vi "Autonomous Independent.vi"   [LabVIEW 2013]
doc: "This VI is called when autonomous begins, and will automatically be terminated when autonomous ends. You can carry out timed or sensor driven robot movement independently without needing to return to the caller."
uses:
  <vilib>/Rock Robotics/WPI/Solenoid/WPI_SolenoidValue.ctl
  Robot Global Data.vi
  <vilib>/Rock Robotics/WPI/RobotDrive/WPI_RobotDriveGetSetRefNum.vi
  <vilib>/Rock Robotics/WPI/Solenoid/WPI_SolenoidSetEnum.vi
  <vilib>/Rock Robotics/WPI/RobotDrive/WPI_RobotDriveArcadeDrive_Standard(NoSaturation).vi
  <vilib>/Rock Robotics/WPI/Solenoid/Deprecated/WPI_SolenoidGetBool.vi
  <vilib>/Rock Robotics/WPI/Joystick/WPI_JoystickGetSetRefNum.vi
panel:
  # "Be sure to right-click and choose Data Operations>>Make Current Value default if you want to save the array values with the VI"
types:
  T1 = typedef "WPI_JoystickDevRef.ctl" = cluster{"Device":T2}
  T2 = typedef "WPI_JoystickDeviceEnum.ctl" = enum16{"USB 1", "USB 2", "USB 3", "USB 4", "Kinect 1", "Kinect 2"}
  T3 = typedef "WPI_MotorControlDeviceRef.ctl" = cluster{"DeviceStatus":errorcluster, "Type":enum16{"PWM", "CAN"}, "PWM":cluster{"Digital Module":T4, "PWM Channel":T5, "DeadBand":T6}, "CAN":cluster{"Device Number":u8, "Control Mode":T7, "Semaphore":T8, "Max Vout":dbl}, "Invert":bool, "TransformRef":T9, "InvTransformRef":T9}
  T4 = typedef "FPGA_TypedefDigitalModule.ctl" = enum16{"Digital Module 1", "Digital Module 2"}
  T5 = typedef "FPGA_DIOPWMChannel.ctl" = enum8{"PWM 1", "PWM 2", "PWM 3", "PWM 4", "PWM 5", "PWM 6", "PWM 7", "PWM 8", "PWM 9", "PWM 10", "Invalid"}
  T6 = typedef "WPI_PWMDeadband.ctl" = cluster{"Name":string, "maxPositivePwm":i32, "minPositivePwm":i32, "centerPwm":i32, "maxNegativePwm":i32, "minNegativePwm":i32, "angularRange":u16}
  T7 = typedef "WPI_CANJaguar_ControlMode.ctl" = enum8{"Percent VBus", "Current", "Speed", "Position", "Voltage"}
  T8 = typedef "Semaphore RefNum" = refnum<k1>
  T9 = typedef "WPI_PWMTransform_ConPane.ctl" = refnum<vi>
  T10 = typedef "WPI_RobotDriveDevRef.ctl" = cluster{"DevStatus":errorcluster, "Motors[]":T3[], "Square Inputs":bool, "Max Output":dbl, "Isochronous":bool}
  T11 = typedef "WPI_SolenoidDevRef.ctl" = cluster{"DevStatus":errorcluster, "Solenoid Module":T12, "Forward Solenoid Channel":T13, "Reverse Solenoid Channel":T13}
  T12 = typedef "FPGA_TypedefSolenoidModule.ctl" = enum16{"Solenoid Module 1", "Solenoid Module 2"}
  T13 = typedef "WPI_SolenoidChannel.ctl" = enum8{"Solenoid 1", "Solenoid 2", "Solenoid 3", "Solenoid 4", "Solenoid 5", "Solenoid 6", "Solenoid 7", "Solenoid 8", "Invalid"}
  T14 = cluster{"axis 1 (x)":dbl, "axis 2 (y)":dbl, "axis 3 (throttle)":dbl, "axis 4":dbl, "axis 5":dbl, "axis 6":dbl}
  T15 = typedef "WPI_SolenoidValue.ctl" = enum16{"Off", "On", "Forward", "Reverse"}
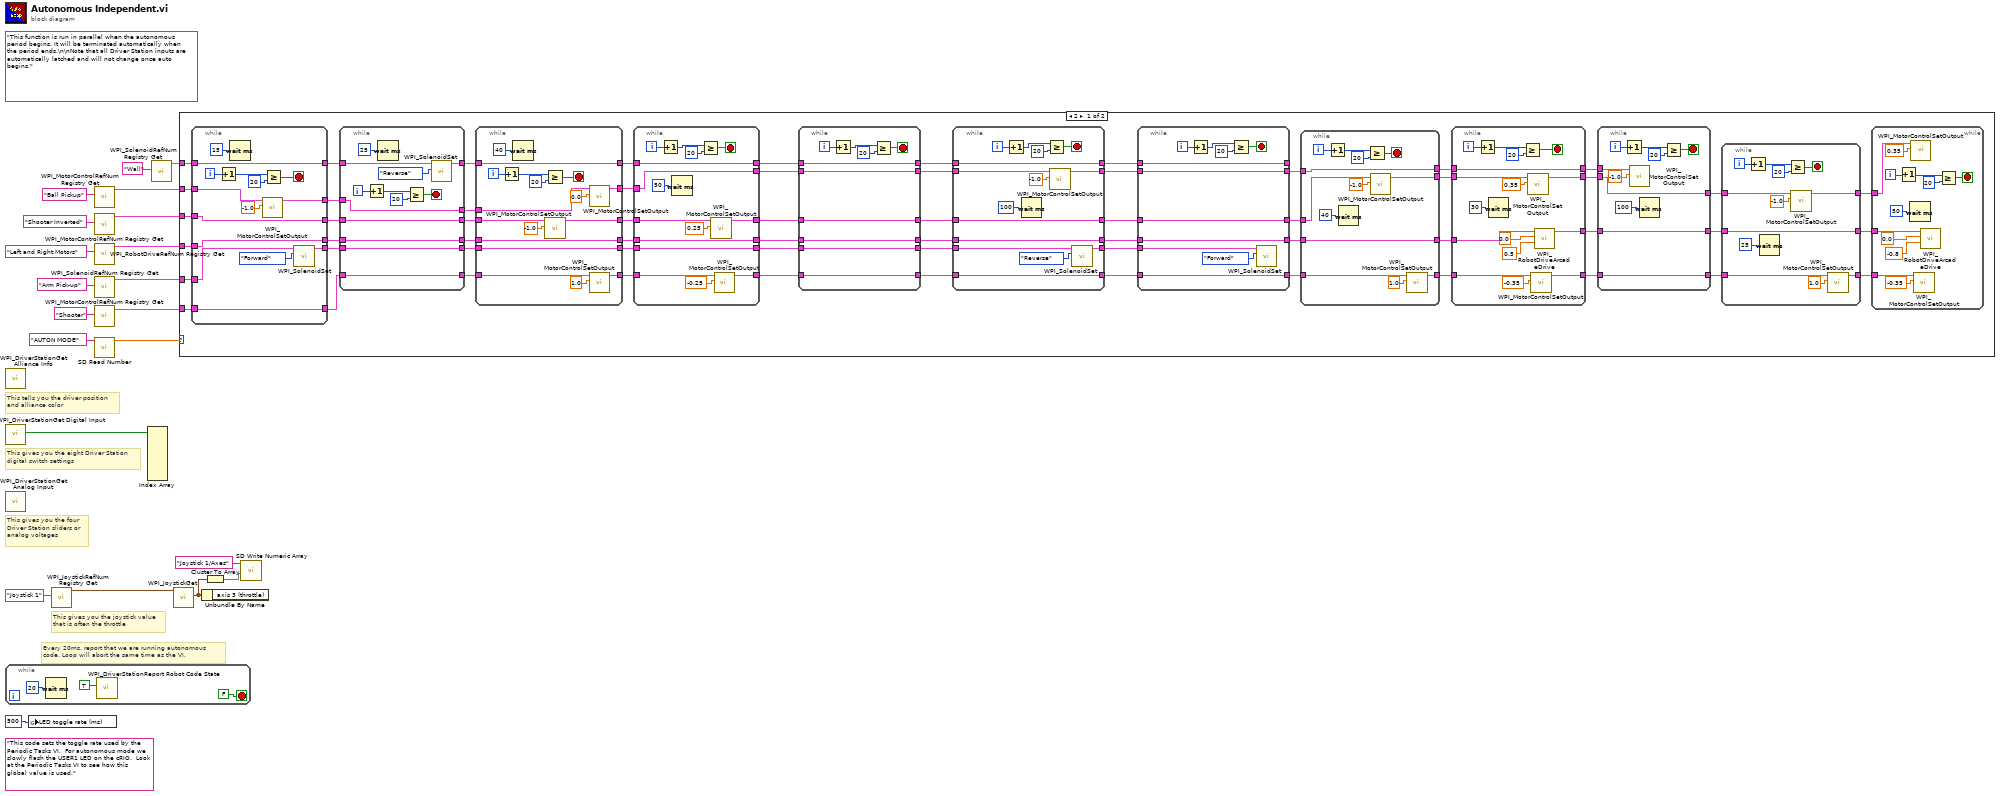
[diagram p0: block diagram]
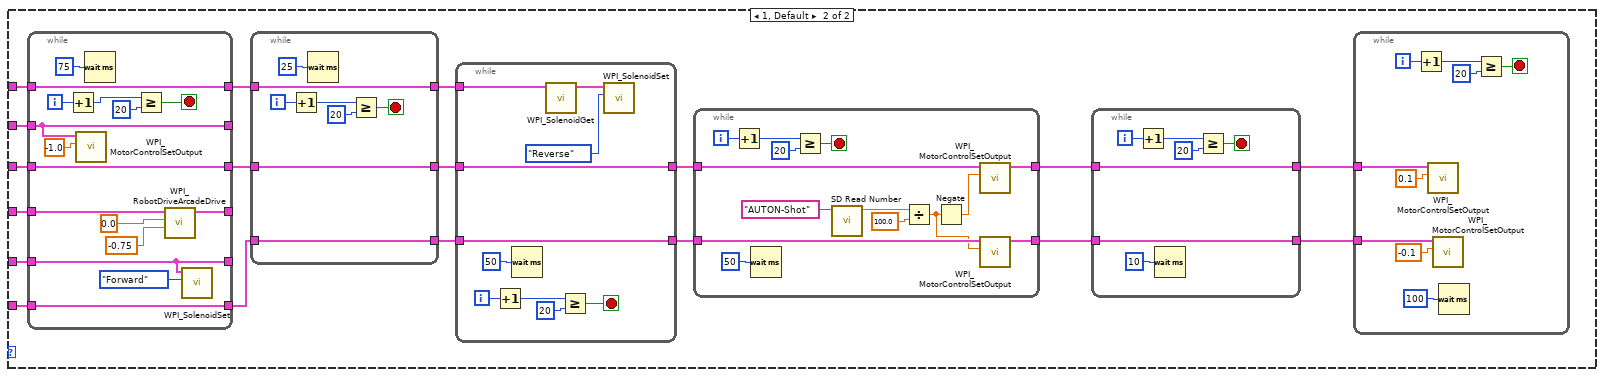
[diagram p2: hidden frame]
diagram:
  (unwired) "This code sets the toggle rate used by the Periodic Tasks VI.  For autonomous mode we slowly flash the USER1 LED on the cRIO.  Look at the Periodic Tasks VI to see how this global value is used."
  (unwired) "This function is run in parallel when the autonomous period begins. It will be terminated automatically when the period ends.\n\nNote that all Driver Station inputs are automatically latched and will not change once auto begins."
  # "Every 20ms, report that we are running autonomous\ncode. Loop will abort the same time as the VI."
  # "This gives you the joystick value\nthat is often the throttle"
  # "This tells you the driver position\nand alliance color"
  # "This gives you the eight Driver Station\ndigital switch settings"
  # "This gives you the four\nDriver Station sliders or\nanalog voltages"
  n1 = call <vilib>:"WPI_DriverStationGet Alliance Info.vi"() -> ()  [unwired: 12 out]
  n2 = call <vilib>:"WPI_DriverStationGet Digital Input.vi"() -> ("Driver Station Digital Input (1-8)"=w21:bool[])  [unwired: 11 out]
  n3 = call <vilib>:"WPI_DriverStationGet Analog Input.vi"() -> ()  [unwired: 12 out]
  n4 = while {
    stop <- FALSE stop-if-true
    n5 = Wait (ms)(milliseconds to wait=u32 20) -> ()  [unwired: 1 out]
    n6 = call <vilib>:"WPI_DriverStationReport Robot Code State.vi"("Autonomous"=TRUE) -> ()  [unwired: 10 in, 1 out]
  }
  n7 = global write "Robot Global Data.vi" "LED toggle rate (ms)"(u32 500 ("LED ms toggle rate")) -> ()
  n8 = call <vilib>:"WPI_JoystickRefNum Registry Get.vi"("refnum name"="Joystick 1") -> ("JoystickDevRef"=w19:T1)  [unwired: 1 in, 9 out]
  n9 = call <vilib>:"WPI_MotorControlRefNum Registry Get.vi"("refnum name"="Ball Pickup") -> ("MotorControlDevRef"=w1:T3)  [unwired: 9 in, 1 out]
  n10 = call <vilib>:"WPI_MotorControlRefNum Registry Get.vi"("refnum name"="Shooter Inverted") -> ("MotorControlDevRef"=w3:T3)  [unwired: 9 in, 1 out]
  n11 = call <vilib>:"WPI_RobotDriveRefNum Registry Get.vi"("refnum name"="Left and Right Motors") -> ("RobotDriveDevRef"=w6:T10)  [unwired: 9 in, 1 out]
  n12 = call <vilib>:"WPI_SolenoidRefNum Registry Get.vi"("refnum name"="Arm Pick-up") -> ("SolenoidDevRef"=w2:T11)  [unwired: 9 in, 1 out]
  n13 = call <vilib>:"WPI_MotorControlRefNum Registry Get.vi"("refnum name"="Shooter") -> ("MotorControlDevRef"=w4:T3)  [unwired: 9 in, 1 out]
  n14 = call <vilib>:"SD Read Number.vi"("Name"="AUTON MODE") -> ("Numeric"=w13:dbl)  [unwired: 8 in, 2 out]
  n15 = Index Array(array=w21) -> ()  [unwired: 8 in, 8 out]
  n16 = call <vilib>:"WPI_SolenoidRefNum Registry Get.vi"("refnum name"="Wall") -> ("SolenoidDevRef"=w5:T11)  [unwired: 9 in, 1 out]
  n17 = call <vilib>:"WPI_JoystickGet.vi"("JoystickDevRef"=w19) -> ("Axes"=w16:T14)  [unwired: 1 in, 5 out]
  n18 = case shown="2" w13 {
    tunnel: w6 -> [w83 w261]
    tunnel: w5 -> [w84 w250]
    tunnel: w4 -> [w82 w260]
    tunnel: w3 -> [w81 w259]
    tunnel: w2 -> [w80 w258]
    tunnel: w1 -> [w79 w257]
    frame 2 {
      n19 = while {
        tunnel: w84 -> [w239]
        tunnel: [w239] -> w74
        tunnel: w83 -> [w236]
        tunnel: [w238] -> w76
        tunnel: w82 -> [w238]
        tunnel: w81 -> [w237]
        tunnel: [w237] -> w77
        tunnel: w80 -> [w231]
        tunnel: w79 -> [w234]
        tunnel: [w236] -> w75
        tunnel: [w233] -> w78
        tunnel: [w229] -> w26
        i -> [w243]
        stop <- w241 stop-if-true
        n20 = Increment(x=w243) -> (x+1=w242:i32)
        n21 = Wait (ms)(milliseconds to wait=u32 15) -> ()  [unwired: 1 out]
        n22 = call <vilib>:"WPI_MotorControlSetOutput.vi"("Output"=-1.0, "MotorControlDevRef"=w234) -> ("MotorControlDevRef"=w233:T3)  [unwired: 7 in, 2 out]
        n23 = Greater Or Equal?(x=w242, y=20) -> (x >= y?=w241:bool)
        n24 = call-poly <vilib>:"WPI_SolenoidSet.vi"("Value"=WPI_SolenoidValue."Forward", "SolenoidDevRef"=w231) -> ("SolenoidDevRef"=w229:T11)  [unwired: 8 in, 1 out]
      }
      n25 = while {
        tunnel: w78 -> [w219]
        tunnel: w77 -> [w220]
        tunnel: w76 -> [w221]
        tunnel: w75 -> [w222]
        tunnel: w74 -> [w224]
        tunnel: [w222] -> w73
        tunnel: [w221] -> w72
        tunnel: [w220] -> w71
        tunnel: [w219] -> w70
        tunnel: [w218] -> w69
        tunnel: [w216] -> w27
        tunnel: w26 -> [w216]
        i -> [w226]
        stop <- w225 stop-if-true
        n26 = Increment(x=w226) -> (x+1=w227:i32)
        n27 = Wait (ms)(milliseconds to wait=u32 25) -> ()  [unwired: 1 out]
        n28 = Greater Or Equal?(x=w227, y=20) -> (x >= y?=w225:bool)
        n29 = call-poly <vilib>:"WPI_SolenoidSet.vi"("Value"=WPI_SolenoidValue."Reverse", "SolenoidDevRef"=w224) -> ("SolenoidDevRef"=w218:T11)  [unwired: 8 in, 1 out]
      }
      n30 = while {
        tunnel: w73 -> [w207]
        tunnel: w72 -> [w210]
        tunnel: w71 -> [w211]
        tunnel: w70 -> [w202]
        tunnel: [w201] -> w64
        tunnel: [w207] -> w67
        tunnel: [w206] -> w68
        tunnel: w69 -> [w206]
        tunnel: [w205] -> w66
        tunnel: [w204] -> w65
        tunnel: [w199] -> w28
        tunnel: w27 -> [w199]
        i -> [w212]
        stop <- w213 stop-if-true
        n31 = Increment(x=w212) -> (x+1=w215:i32)
        n32 = Wait (ms)(milliseconds to wait=u32 40) -> ()  [unwired: 1 out]
        n33 = Greater Or Equal?(x=w215, y=20) -> (x >= y?=w213:bool)
        n34 = call <vilib>:"WPI_MotorControlSetOutput.vi"("Output"=-1.0, "MotorControlDevRef"=w211) -> ("MotorControlDevRef"=w204:T3)  [unwired: 7 in, 2 out]
        n35 = call <vilib>:"WPI_MotorControlSetOutput.vi"("Output"=0.0, "MotorControlDevRef"=w202) -> ("MotorControlDevRef"=w201:T3)  [unwired: 7 in, 2 out]
        n36 = call <vilib>:"WPI_MotorControlSetOutput.vi"("Output"=1.0, "MotorControlDevRef"=w210) -> ("MotorControlDevRef"=w205:T3)  [unwired: 7 in, 2 out]
      }
      n37 = while {
        tunnel: w68 -> [w186]
        tunnel: w67 -> [w187]
        tunnel: w66 -> [w197]
        tunnel: w65 -> [w198]
        tunnel: w64 -> [w185]
        tunnel: [w189] -> w61
        tunnel: [w188] -> w60
        tunnel: [w187] -> w62
        tunnel: [w186] -> w63
        tunnel: [w185] -> w59
        tunnel: [w184] -> w29
        tunnel: w28 -> [w184]
        i -> [w192]
        stop <- w191 stop-if-true
        n38 = Increment(x=w192) -> (x+1=w193:i32)
        n39 = Wait (ms)(milliseconds to wait=u32 50) -> ()  [unwired: 1 out]
        n40 = Greater Or Equal?(x=w193, y=20) -> (x >= y?=w191:bool)
        n41 = call <vilib>:"WPI_MotorControlSetOutput.vi"("Output"=0.25, "MotorControlDevRef"=w198) -> ("MotorControlDevRef"=w188:T3)  [unwired: 7 in, 2 out]
        n42 = call <vilib>:"WPI_MotorControlSetOutput.vi"("Output"=-0.25, "MotorControlDevRef"=w197) -> ("MotorControlDevRef"=w189:T3)  [unwired: 7 in, 2 out]
      }
      n43 = while {
        tunnel: w63 -> [w175]
        tunnel: w62 -> [w176]
        tunnel: w61 -> [w179]
        tunnel: w60 -> [w178]
        tunnel: w59 -> [w177]
        tunnel: [w179] -> w55
        tunnel: [w178] -> w54
        tunnel: [w177] -> w58
        tunnel: [w176] -> w56
        tunnel: [w175] -> w57
        tunnel: [w174] -> w30
        tunnel: w29 -> [w174]
        i -> [w181]
        stop <- w180 stop-if-true
        n44 = Increment(x=w181) -> (x+1=w183:i32)
        n45 = Greater Or Equal?(x=w183, y=20) -> (x >= y?=w180:bool)
      }
      n46 = while {
        tunnel: w58 -> [w169]
        tunnel: [w167] -> w49
        tunnel: w57 -> [w167]
        tunnel: [w166] -> w50
        tunnel: w56 -> [w166]
        tunnel: [w165] -> w51
        tunnel: w55 -> [w165]
        tunnel: [w164] -> w52
        tunnel: w54 -> [w164]
        tunnel: [w162] -> w42
        tunnel: w30 -> [w161]
        tunnel: [w159] -> w25
        i -> [w171]
        stop <- w170 stop-if-true
        n47 = Increment(x=w171) -> (x+1=w172:i32)
        n48 = Wait (ms)(milliseconds to wait=u32 100) -> ()  [unwired: 1 out]
        n49 = Greater Or Equal?(x=w172, y=20) -> (x >= y?=w170:bool)
        n50 = call <vilib>:"WPI_MotorControlSetOutput.vi"("Output"=-1.0, "MotorControlDevRef"=w169) -> ("MotorControlDevRef"=w162:T3)  [unwired: 7 in, 2 out]
        n51 = call-poly <vilib>:"WPI_SolenoidSet.vi"("Value"=WPI_SolenoidValue."Reverse", "SolenoidDevRef"=w161) -> ("SolenoidDevRef"=w159:T11)  [unwired: 8 in, 1 out]
      }
      n52 = while {
        tunnel: w49 -> [w126]
        tunnel: w50 -> [w127]
        tunnel: w51 -> [w129]
        tunnel: w52 -> [w128]
        tunnel: [w129] -> w47
        tunnel: [w128] -> w53
        tunnel: [w127] -> w48
        tunnel: [w126] -> _
        tunnel: [w125] -> w39
        tunnel: w42 -> [w125]
        tunnel: w25 -> [w124]
        i -> [w131]
        stop <- w130 stop-if-true
        n53 = Increment(x=w131) -> (x+1=w133:i32)
        n54 = Greater Or Equal?(x=w133, y=20) -> (x >= y?=w130:bool)
        n55 = call-poly <vilib>:"WPI_SolenoidSet.vi"("Value"=WPI_SolenoidValue."Forward", "SolenoidDevRef"=w124) -> ()  [unwired: 8 in, 2 out]
      }
      n56 = while {
        tunnel: w53 -> [w153]
        tunnel: w47 -> [w154]
        tunnel: w48 -> [w150]
        tunnel: [w150] -> w46
        tunnel: [w149] -> w45
        tunnel: [w148] -> w44
        tunnel: [w146] -> w40
        tunnel: w39 -> [w146]
        i -> [w155]
        stop <- w156 stop-if-true
        n57 = Increment(x=w155) -> (x+1=w158:i32)
        n58 = Wait (ms)(milliseconds to wait=u32 40) -> ()  [unwired: 1 out]
        n59 = Greater Or Equal?(x=w158, y=20) -> (x >= y?=w156:bool)
        n60 = call <vilib>:"WPI_MotorControlSetOutput.vi"("Output"=-1.0, "MotorControlDevRef"=w153) -> ("MotorControlDevRef"=w148:T3)  [unwired: 7 in, 2 out]
        n61 = call <vilib>:"WPI_MotorControlSetOutput.vi"("Output"=1.0, "MotorControlDevRef"=w154) -> ("MotorControlDevRef"=w149:T3)  [unwired: 7 in, 2 out]
      }
      n62 = while {
        tunnel: w46 -> [w118]
        tunnel: w45 -> [w112]
        tunnel: w44 -> [w110]
        tunnel: [w111] -> w37
        tunnel: [w109] -> w38
        tunnel: [w114] -> w43
        tunnel: [w113] -> w41
        tunnel: w40 -> [w113]
        i -> [w119]
        stop <- w120 stop-if-true
        n63 = Increment(x=w119) -> (x+1=w121:i32)
        n64 = Wait (ms)(milliseconds to wait=u32 30) -> ()  [unwired: 1 out]
        n65 = Greater Or Equal?(x=w121, y=20) -> (x >= y?=w120:bool)
        n66 = call <vilib>:"WPI_MotorControlSetOutput.vi"("Output"=0.35, "MotorControlDevRef"=w110) -> ("MotorControlDevRef"=w109:T3)  [unwired: 7 in, 2 out]
        n67 = call <vilib>:"WPI_MotorControlSetOutput.vi"("Output"=-0.35, "MotorControlDevRef"=w112) -> ("MotorControlDevRef"=w111:T3)  [unwired: 7 in, 2 out]
        n68 = call-poly <vilib>:"WPI_RobotDriveArcadeDrive.vi"("Y axis value"=0.5, "X axis value"=0.0, "RobotDriveDevRef"=w118) -> ("RobotDriveDevRef"=w114:T10)  [unwired: 6 in, 2 out]
      }
      n69 = while {
        tunnel: w43 -> [w98]
        tunnel: w41 -> [w102]
        tunnel: w38 -> [w100]
        tunnel: [w100] -> w35
        tunnel: w37 -> [w99]
        tunnel: [w99] -> w36
        tunnel: [w98] -> w34
        i -> [w103]
        stop <- w104 stop-if-true
        n70 = Increment(x=w103) -> (x+1=w106:i32)
        n71 = call <vilib>:"WPI_MotorControlSetOutput.vi"("Output"=-1.0, "MotorControlDevRef"=w102) -> ()  [unwired: 7 in, 3 out]
        n72 = Wait (ms)(milliseconds to wait=u32 100) -> ()  [unwired: 1 out]
        n73 = Greater Or Equal?(x=w106, y=20) -> (x >= y?=w104:bool)
      }
      n74 = while {
        tunnel: w36 -> [w91]
        tunnel: w35 -> [w89]
        tunnel: [w92] -> w33
        tunnel: w34 -> [w92]
        tunnel: [w90] -> w32
        tunnel: [w88] -> w31
        i -> [w94]
        stop <- w93 stop-if-true
        n75 = Increment(x=w94) -> (x+1=w95:i32)
        n76 = Wait (ms)(milliseconds to wait=u32 25) -> ()  [unwired: 1 out]
        n77 = Greater Or Equal?(x=w95, y=20) -> (x >= y?=w93:bool)
        n78 = call <vilib>:"WPI_MotorControlSetOutput.vi"("Output"=-1.0, "MotorControlDevRef"=w89) -> ("MotorControlDevRef"=w88:T3)  [unwired: 7 in, 2 out]
        n79 = call <vilib>:"WPI_MotorControlSetOutput.vi"("Output"=1.0, "MotorControlDevRef"=w91) -> ("MotorControlDevRef"=w90:T3)  [unwired: 7 in, 2 out]
      }
      n80 = while {
        tunnel: w33 -> [w143]
        tunnel: w32 -> [w145]
        tunnel: w31 -> [w144]
        i -> [w135]
        stop <- w136 stop-if-true
        n81 = Increment(x=w135) -> (x+1=w137:i32)
        n82 = Wait (ms)(milliseconds to wait=u32 50) -> ()  [unwired: 1 out]
        n83 = call <vilib>:"WPI_MotorControlSetOutput.vi"("Output"=0.35, "MotorControlDevRef"=w144) -> ()  [unwired: 7 in, 3 out]
        n84 = call <vilib>:"WPI_MotorControlSetOutput.vi"("Output"=-0.35, "MotorControlDevRef"=w145) -> ()  [unwired: 7 in, 3 out]
        n85 = call-poly <vilib>:"WPI_RobotDriveArcadeDrive.vi"("Y axis value"=-0.8, "X axis value"=0.0, "RobotDriveDevRef"=w143) -> ()  [unwired: 6 in, 3 out]
        n86 = Greater Or Equal?(x=w137, y=20) -> (x >= y?=w136:bool)
      }
    }
    frame 1, Default {
      n87 = while {
        tunnel: w261 -> [w321]
        tunnel: [w319] -> _
        tunnel: [w318] -> w247
        tunnel: w260 -> [w318]
        tunnel: w259 -> [w317]
        tunnel: [w317] -> w244
        tunnel: w258 -> [w312]
        tunnel: w257 -> [w311]
        tunnel: [w311] -> _
        tunnel: [w312] -> _
        tunnel: [w314] -> w249
        tunnel: w250 -> [w314]
        i -> [w325]
        stop <- w322 stop-if-true
        n88 = Increment(x=w325) -> (x+1=w324:i32)
        n89 = call <vilib>:"WPI_MotorControlSetOutput.vi"("Output"=-1.0, "MotorControlDevRef"=w311) -> ()  [unwired: 7 in, 3 out]
        n90 = Wait (ms)(milliseconds to wait=u32 75) -> ()  [unwired: 1 out]
        n91 = Greater Or Equal?(x=w324, y=20) -> (x >= y?=w322:bool)
        n92 = call-poly <vilib>:"WPI_RobotDriveArcadeDrive.vi"("Y axis value"=-0.75, "X axis value"=0.0, "RobotDriveDevRef"=w321) -> ("RobotDriveDevRef"=w319:T10)  [unwired: 6 in, 2 out]
        n93 = call-poly <vilib>:"WPI_SolenoidSet.vi"("Value"=WPI_SolenoidValue."Forward", "SolenoidDevRef"=w312) -> ()  [unwired: 8 in, 2 out]
      }
      n94 = while {
        tunnel: w249 -> [w269]
        tunnel: [w269] -> w248
        tunnel: w247 -> [w268]
        tunnel: [w268] -> w246
        tunnel: [w267] -> w245
        tunnel: w244 -> [w267]
        i -> [w264]
        stop <- w263 stop-if-true
        n95 = Increment(x=w264) -> (x+1=w265:i32)
        n96 = Wait (ms)(milliseconds to wait=u32 25) -> ()  [unwired: 1 out]
        n97 = Greater Or Equal?(x=w265, y=20) -> (x >= y?=w263:bool)
      }
      n98 = while {
        tunnel: w246 -> [w304]
        tunnel: w245 -> [w305]
        tunnel: [w305] -> w256
        tunnel: [w304] -> w255
        tunnel: w248 -> [w302]
        i -> [w307]
        stop <- w306 stop-if-true
        n99 = Increment(x=w307) -> (x+1=w308:i32)
        n100 = Wait (ms)(milliseconds to wait=u32 50) -> ()  [unwired: 1 out]
        n101 = call-poly <vilib>:"WPI_SolenoidGet.vi"("SolenoidDevRef"=w302) -> ("SolenoidDevRef"=w300:T11)  [unwired: 8 in, 2 out]
        n102 = Greater Or Equal?(x=w308, y=20) -> (x >= y?=w306:bool)
        n103 = call-poly <vilib>:"WPI_SolenoidSet.vi"("Value"=WPI_SolenoidValue."Reverse", "SolenoidDevRef"=w300) -> ()  [unwired: 8 in, 2 out]
      }
      n104 = while {
        tunnel: w256 -> [w295]
        tunnel: w255 -> [w294]
        tunnel: [w293] -> w254
        tunnel: [w292] -> w253
        i -> [w297]
        stop <- w296 stop-if-true
        n105 = Increment(x=w297) -> (x+1=w299:i32)
        n106 = Wait (ms)(milliseconds to wait=u32 50) -> ()  [unwired: 1 out]
        n107 = Greater Or Equal?(x=w299, y=20) -> (x >= y?=w296:bool)
        n108 = call <vilib>:"SD Read Number.vi"("Name"="AUTON-Shot") -> ("Numeric"=w288:dbl)  [unwired: 8 in, 2 out]
        n109 = Divide(x=w288, y=100.0) -> (x/y=w287:dbl)
        n110 = Negate(x=w287) -> (-x=w289:dbl)
        n111 = call <vilib>:"WPI_MotorControlSetOutput.vi"("Output"=w289, "MotorControlDevRef"=w295) -> ("MotorControlDevRef"=w292:T3)  [unwired: 7 in, 2 out]
        n112 = call <vilib>:"WPI_MotorControlSetOutput.vi"("Output"=w287, "MotorControlDevRef"=w294) -> ("MotorControlDevRef"=w293:T3)  [unwired: 7 in, 2 out]
      }
      n113 = while {
        tunnel: w254 -> [w281]
        tunnel: w253 -> [w280]
        tunnel: [w281] -> w251
        tunnel: [w280] -> w252
        i -> [w282]
        stop <- w283 stop-if-true
        n114 = Increment(x=w282) -> (x+1=w284:i32)
        n115 = Wait (ms)(milliseconds to wait=u32 10) -> ()  [unwired: 1 out]
        n116 = Greater Or Equal?(x=w284, y=20) -> (x >= y?=w283:bool)
      }
      n117 = while {
        tunnel: w252 -> [w277]
        tunnel: w251 -> [w278]
        i -> [w272]
        stop <- w271 stop-if-true
        n118 = Increment(x=w272) -> (x+1=w274:i32)
        n119 = call <vilib>:"WPI_MotorControlSetOutput.vi"("Output"=0.1, "MotorControlDevRef"=w277) -> ()  [unwired: 7 in, 3 out]
        n120 = call <vilib>:"WPI_MotorControlSetOutput.vi"("Output"=-0.1, "MotorControlDevRef"=w278) -> ()  [unwired: 7 in, 3 out]
        n121 = Wait (ms)(milliseconds to wait=u32 100) -> ()  [unwired: 1 out]
        n122 = Greater Or Equal?(x=w274, y=20) -> (x >= y?=w271:bool)
      }
    }
  }
  n123 = Unbundle By Name(w16) -> ()  [unwired: 1 out]
  n124 = Cluster To Array(cluster=w16) -> (array=w17:dbl[])
  n125 = call <vilib>:"SD Write Numeric Array.vi"("Numeric Array"=w17, "Name"="Joystick 1/Axes") -> ()  [unwired: 8 in, 2 out]
